vi "CRYGet LocalInfo.vi"() -> ()   [LabVIEW 2013]
uses:
  Kernel32.DLL
panel:
  in  "String":string="12345678"
  out "LCDData":string
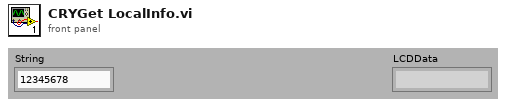
[diagram p1: front panel]
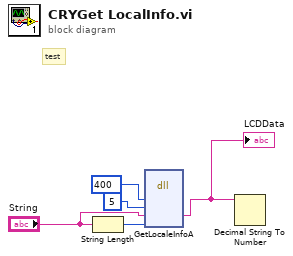
[diagram p0: block diagram]
diagram:
  # "test"
  n1 = String Length(string="String") -> (length=w2:i32)
  n2 = dll-call lib="kernel32.dll" fn="GetLocaleInfoA" label="GetACP()"("LocalId"=u32 400, "LCType"=u32 5 ("LocalId"), "LCDData"="String", "Size"=w2) -> ("LCDData"=w3:string)  [unwired: 3 in, 6 out]
  "LCDData" <- w3
  n3 = Decimal String To Number(string=w3) -> ()  [unwired: 2 in, 2 out]
